vi "GetYearList.vi"() -> (3 "Array":string[](array[string]))   [LabVIEW 2013, in "UI_TimeSelector.xctl"]
uses:
  UI_TimeSelector/UI_TimeSelector.xctl
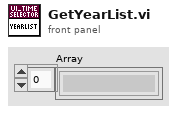
[diagram p1: front panel]
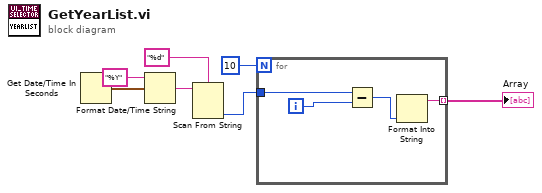
[diagram p0: block diagram]
diagram:
  n1 = Get Date/Time In Seconds() -> (seconds since 1Jan1904=w1:timestamp)
  n2 = Format Date/Time String(time format string (%c)="%Y", seconds (now)=w1) -> (date/time string=w3:string)  [unwired: 1 in]
  n3 = Scan From String(format string="%d", input string=w3) -> (output 1=w5:i32)  [unwired: 3 in, 3 out]
  n4 = for {
    N: 10 -> [_]
    tunnel: w5 -> [w11]
    tunnel: [w8] -> w7 mode=indexing
    i -> [w10]
    n5 = Subtract(x=w11, y=w10) -> (x-y=w9:i32)
    n6 = Format Into String(w9) -> (resulting string=w8:string)  [unwired: 3 in, 1 out]
  }
  "Array" <- w7
